vi "Propagate.vi"(8 "error in (no error)":errorcluster, 11 "CNN in":refnum<class "CNN.lvclass">) -> (0 "error out":errorcluster, 3 "CNN out":refnum<class "CNN.lvclass">)   [LabVIEW 2016, in "CNN.lvclass"]
uses:
  CNN.lvclass
  CNN.lvclass/CNN.ctl
  biCNN/Controls/Type of Neuron.ctl
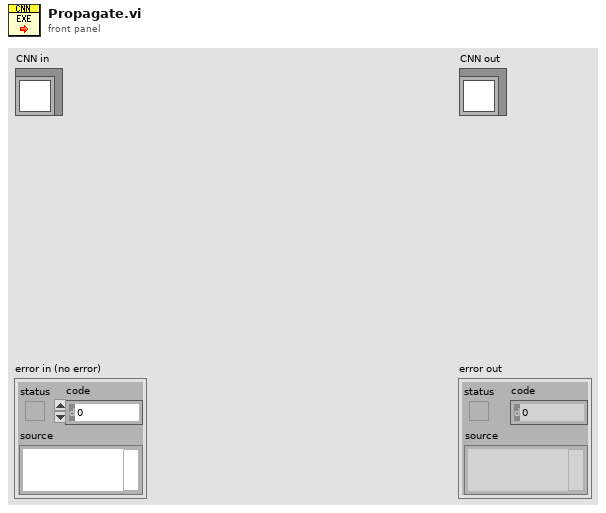
[diagram p1: front panel]
types:
  T1 = typedef "Type of Neuron.ctl" = enum16{"MF", "BA", "GO", "GC", "PC", "LU", "Glia (Dummy)"}
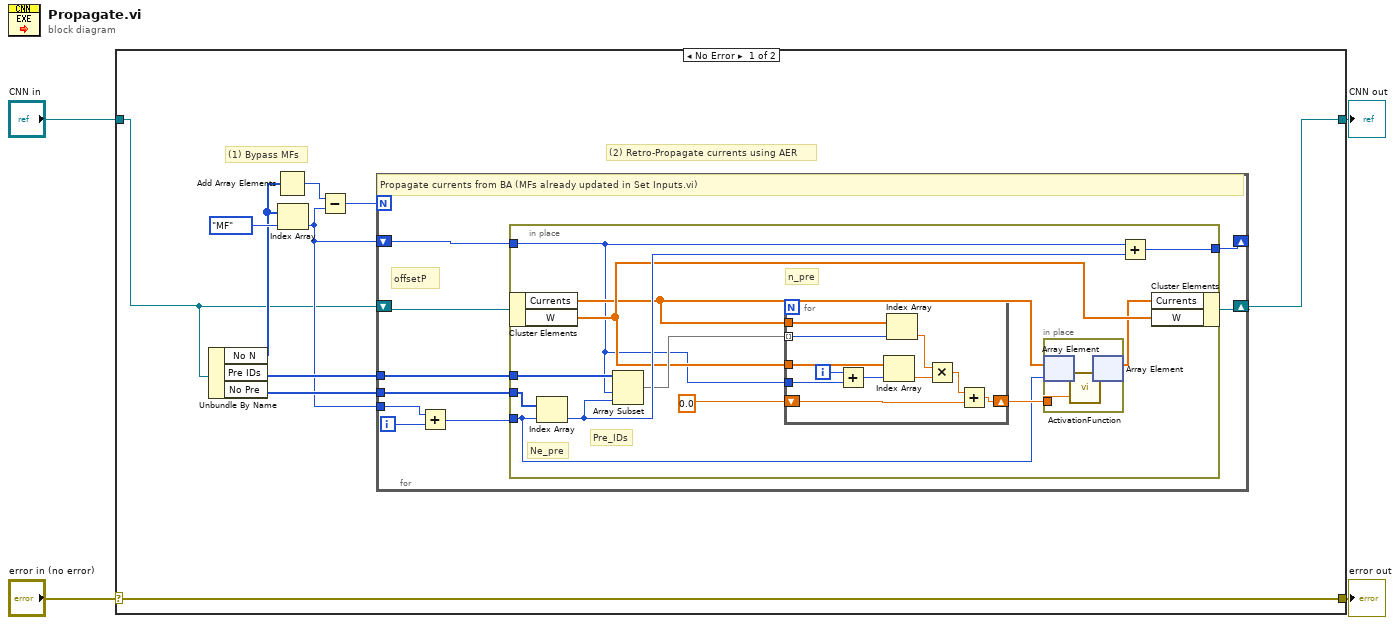
[diagram p0: block diagram]
diagram:
  n1 = case shown="No Error" "error in (no error)" {
    selector: "error in (no error)" -> [w14 w49]
    tunnel: [w14 w49] -> w3
    tunnel: [w5 w50] -> w1
    tunnel: "CNN in" -> [w6 w50]
    frame No Error {
      # "(2) Retro-Propagate currents using AER"
      # "(1) Bypass MFs"
      n2 = Unbundle By Name(w6) -> ("No N"=w10:i32[], "Pre IDs"=w13:i32[], "No Pre"=w12:i32[])
      n3 = Add Array Elements(numeric array=w10) -> (sum=w9:i32)
      n4 = Index Array(array=w10, index=Type_of_Neuron."MF" ("Type of Neuron")) -> (element=w7:i32)
      n5 = Subtract(x=w9, y=w7) -> (x-y=w8:i32)
      n6 = for {
        N: w8 -> [_]
        tunnel: w12 -> [w23]
        shift-right: [w18] -> w5
        shift-left: w6 -> [w19]
        shift-right: [w22] -> _
        shift-left: w7 -> [w20]
        tunnel: w13 -> [w21]
        tunnel: w7 -> [w15]
        i -> [w17]
        # "offsetP"
        # "Propagate currents from BA (MFs already updated in Set Inputs.vi)"
        n7 = Add(x=w15, y=w17) -> (x+y=w16:i32)
        n8 = in-place {
          in-place-border: w23 -> [w34]
          in-place-border: [w33] -> w22
          in-place-border: w21 -> [w32]
          in-place-border: w20 -> [w25]
          in-place-border: w16 -> [w28]
          # "n_pre"
          # "Pre_IDs"
          # "Ne_pre"
          n9 = in-place-cluster #1(w19) -> ("Currents"=w26:dbl[], "W"=w27:dbl[])
          n10 = Index Array(array=w34, index=w28) -> (element=w30:i32)
          n11 = Array Subset(array=w32, index=w25, length=w30) -> (w29:i32[])
          n12 = for {
            shift-right: [w44] -> w35
            shift-left: 0.0 ("N") -> [w46]
            tunnel: w27 -> [w48]
            tunnel: w25 -> [w45]
            tunnel: w29 -> [w38] mode=indexing
            tunnel: w26 -> [w39]
            i -> [w40]
            n13 = Add(x=w40, y=w45) -> (x+y=w43:i32)
            n14 = Index Array(array=w48, index=w43) -> (element=w47:dbl)
            n15 = Index Array(array=w39, index=w38) -> (element=w41:dbl)
            n16 = Multiply(x=w41, y=w47) -> (x*y=w42:dbl)
            n17 = Add(x=w42, y=w46) -> (x+y=w44:dbl)
          }
          n18 = in-place {
            in-place-border: w35 -> [w37]
            n19 = in-place-array #2(w26, w28) -> ()  [unwired: 1 out]
            n20 = call "ActivationFunction.vi"("x"=w37) -> ("y"=w36:dbl)  [unwired: 2 in]
            n21 = in-place-array #2(w36) -> (w24:dbl[])  [unwired: 1 out]
          }
          n22 = Add(x=w25, y=w30) -> (x+y=w33:i32)
          n23 = in-place-cluster #1("Currents"=w24, "W"=w27) -> (w18:refnum<class "CNN.lvclass">)
        }
      }
    }
    frame Error {
    }
  }
  "error out" <- w3
  "CNN out" <- w1
